vi "Dialog window display loop.vi"(1 "Loop ID":T1, 11 "error in (no error)":errorcluster) -> ()   [LabVIEW 2011]
uses:
  Application Structure/Loop ID.ctl
  Application Structure/QSM State List.ctl
  emi cndiates/E&S/reate/S&E Event source.ctl
  Annotation/Annotation Message.ctl
  emi Lib/System 01/0 - General/emi_Read System ID.vi
  emi Lib/System 01/0 - General/App/Loop control 2/Private/_emi_ SMLoop start condition.vi
  emi Lib/System 01/0 - General/App/Loop control 2/Private/_emi_ SMLoop Error Check.vi
  emi Lib/Basic/0 - General/Error/emi_Is Error.vi
  emi Lib/System 01/0 - General/App/Loop control 2/Private/_emi_SMLoop Register new.vi
  emi Lib/System 01/0 - General/S&E reporting/emi_Send S&E Error message.vi
  emi Lib/Basic/0 - General/Error/emi_ Is Error state.vi
  emi Lib/System 01/0 - General/App/Loop control/Private/_emi_GFV Loop Linking.vi
  emi Lib/System 01/0 - General/App/Loop control/Private/_emi_GFV Loop Enable.vi
  emi Lib/System 01/0 - General/App/Loop control 2/Private/_emi_ SMLoop Restart.vi
  emi Lib/System 01/0 - General/App/Private/_emi_GFV App Close.vi
  emi Lib/System 01/0 - General/App/Loop control 2/Private/_emi_ SMLoop Restart Counter.vi
  emi Lib/System 01/0 - General/App/Loop control/Private/_emi_GFV Loop Running.vi
  emi Lib/System 01/0 - General/Private/_emi_GFV System ID.vi
  emi Lib/System 01/0 - General/S&E reporting/Private/_emi_S&E Q Generator.vi
  <vilib>/Utility/error.llb/Clear Errors.vi
  emi Lib/System 01/0 - General/App/Loop control/Private/_emi_GFV stop a loop so it can reset.vi
  emi Lib/System 01/1 - GUI/Profiling Mar-In/Splash & About/Private/emi_Splash&About Screen.vi
  Application Structure/QSM/QSM Q holder.vi
  emi Lib/Basic/0 - General/Time/Private/emi_Time offset holder.vi
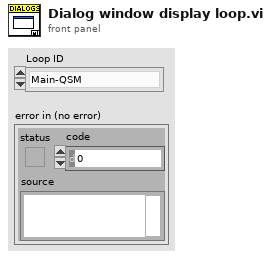
[diagram p1: front panel]
types:
  T1 = typedef "Loop ID.ctl" = enum16{"Main-QSM", "Main-Dialog", "Main-Ind Upd", "Main-Graph Upd", "Main-Debug", "Main-DebugW1", "Main-DebugW2", "Main-SE Handler", "Interface-PCP", "Interface-CANbus", "Interface-Modem", "Var Handling-Beat", "Var Handling-From PCP", "Var Handling-File storage", "Var Handling-From Simulator", "GUI-GrphW Mast", "GUI-GrphW Slav", "SIM-Tool W1", "SIM-Tool W2", "Alm-Sound", "LEIN-motor", "Tool data gatherer Qer", "Tool Data LEIN STAT2 dekoder", "Indicator Value Update", "Tool STAT2 dedicated reader", "Tool ID handler", "Detail View L1", "Detail View L2", "Main display enable view", "Sequence runner", "Voltage setpoint", "Resistance setpoint", "Stroker Wizard L1", "Stroker Wizard L2", "Alarm Handling", "Annotations Tip Strip", "Magna Interface", "Modem Status", "Var Handling - Modem Status", "Power interface detector"}
  T2 = typedef "QSM State List.ctl" = enum16{"Idle", "Init <<<Start>>>", "Init Reg Controlers", "Init Stroker Ref FGV", "Init Driller Ref FGV", "Init Tractor Ref FGV", "Init All loops", "Init Mem Ctls", "Init GUI", "Init<<<End>>>", "Show options", "Options updated", "Show User Dialog", "User Updated", "Show About", "Show Help", "Debug Visibility", "End Application", "Mem Ctls", "Mem Graphs", "Post", "-------------", "Dialog Common Analog", "Chart Init", "Chart Var Selector Rings init", "Chart Read Settings from INI", "Chart Clear", "Chart Selection Changed", "Chart Time Changed", "Graph Dialog Show", "Annotation, New", "Annotation Created", "PCP CMD", "Show Welcome screen", "Dialog Tool analog", "Update PCP resistance", "Tool CMD", "Chart single autoscale", "Tool connenction state", "Show detailed view", "Sequences updated", "Show stroker wizard", "Change tool", "Reset Telemetry", "Update control units", "Stop Logging", "Start New Loggfile", "Log Init", "Copy INI files"}
  T3 = typedef "S&E Event source.ctl" = enum16{"User", "Instrument", "Application", "Windows"}
  T4 = typedef "Annotation Message.ctl" = cluster{"Annotation":string, "User":string, "time":timestamp}
  T5 = typedef "_emi_ SMLoop sates.ctl" = enum16{"Init", "Standby", "Start", "Normal Operation", "Stop", "Error Handling", "End", "Post"}
  T6 = cluster{"Placeholder":bool, "Dialog Selector Q":refnum<queue>}
  T7 = typedef "Dialog selection cluster.ctl" = cluster{"ID":T8, "Details":variant}
  T8 = typedef "Dialog box ID.ctl" = enum16{"About dialog Box", "Options dialog box", "User dialog Box", "Custom dialog...", "Variables Common Analog", "Annotation", "Welcome screen", "Variables Tool Analog", "High G graph display", "Sequence setup", "Unused"}
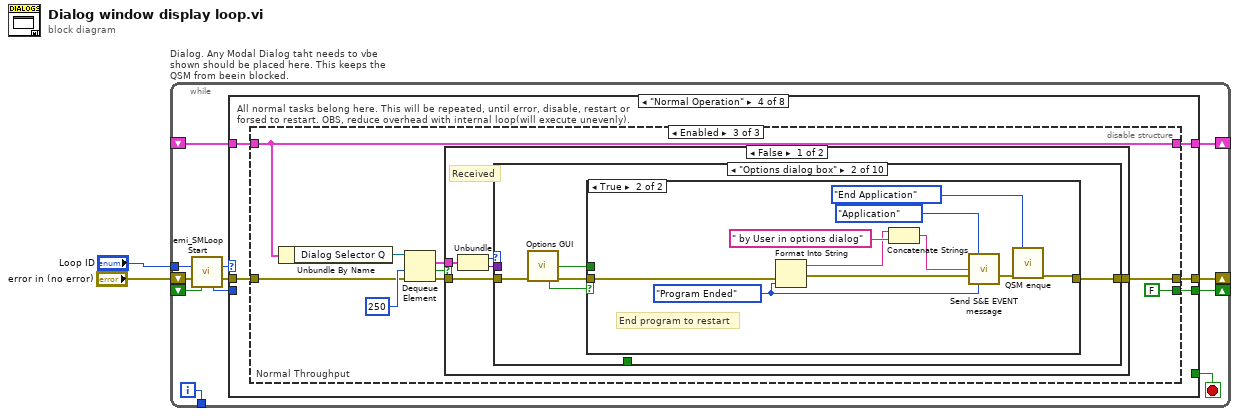
[diagram p0: block diagram]
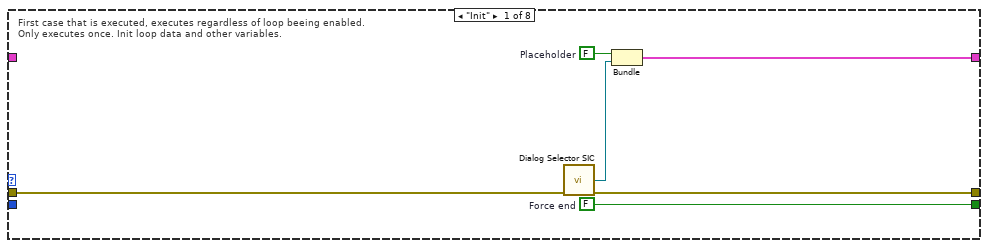
[diagram p2: hidden frame]
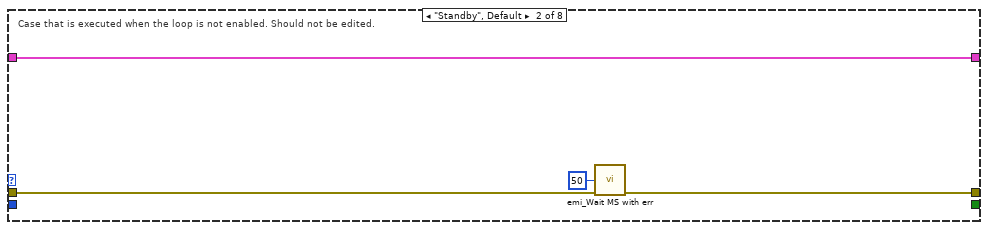
[diagram p3: hidden frame]
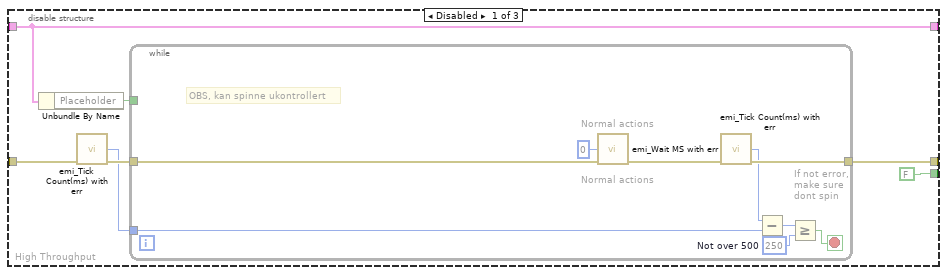
[diagram p5: hidden frame]
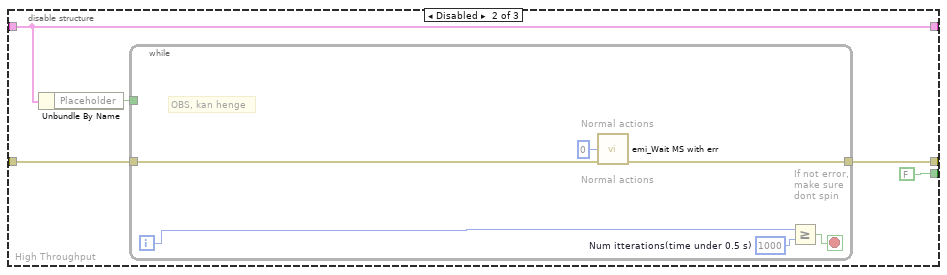
[diagram p6: hidden frame]
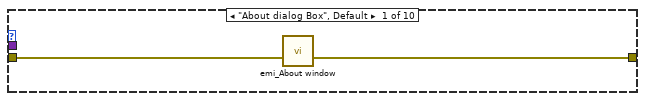
[diagram p7: hidden frame]
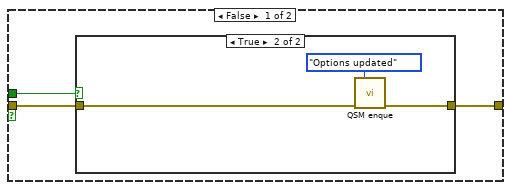
[diagram p8: hidden frame]
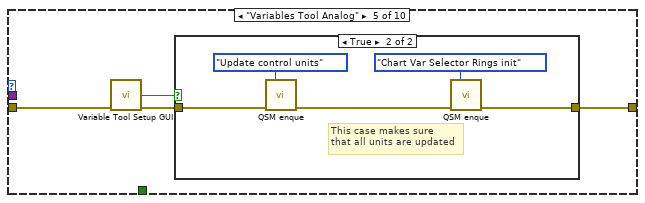
[diagram p12: hidden frame]
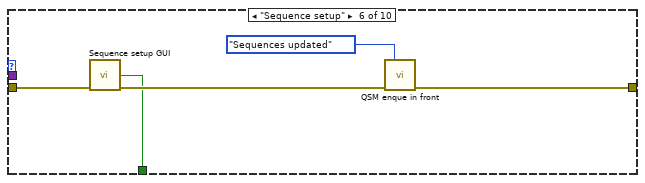
[diagram p14: hidden frame]
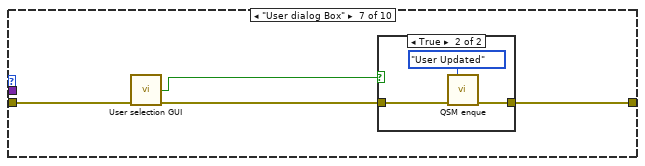
[diagram p15: hidden frame]
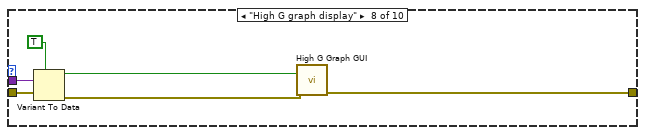
[diagram p17: hidden frame]
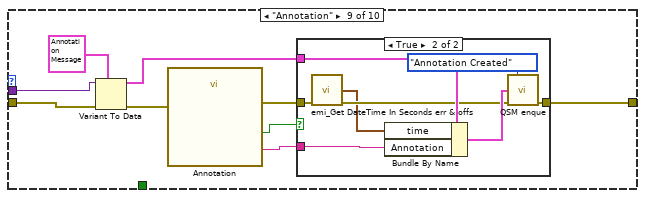
[diagram p18: hidden frame]
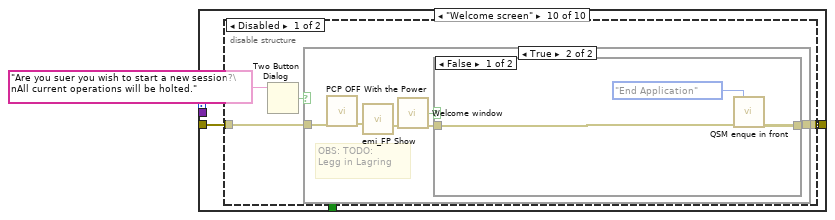
[diagram p20: hidden frame]
diagram:
  n1 = while "Dialog. Any Modal Dialog taht needs to vbe shown should be placed here. This keeps the QSM from beein blocked." {
    shift-right: [w14] -> _
    shift-left: _ -> [w10]
    shift-right: [w12] -> _
    shift-left: "error in (no error)" -> [w8]
    tunnel: [w11] -> _
    shift-right: [w9] -> _
    shift-left: _ -> [w5]
    tunnel: "Loop ID" -> [w6]
    i -> [w11]
    stop <- w13 stop-if-true
    n2 = call "emi_SMLoop Start.vi"("Loop ID"=w6, "error in (no error)"=w8, "Force Stop(F)"=w5) -> ("Loop command"=w4:T5, "error out"=w7:errorcluster, "Loop ID out"=w3:i32)  [unwired: 10 in]
    n3 = case shown="\"Normal Operation\"" w4 {
      tunnel: [w20 w21 w25 w29 w181 w184 w185 w188] -> w14
      tunnel: [_ _ _ _ _ _ _ TRUE] -> w13
      tunnel: w7 -> [w17 w23 w26 w31 w182 w183 w186 w189]
      tunnel: [w16 w22 w26 w30 w182 w183 w186 w189] -> w12
      tunnel: w10 -> [_ w21 w25 w28 w181 w184 w185 w188]
      tunnel: [w18 _ _ w27 _ _ _ _] -> w9
      tunnel: w3 -> [_ _ _ _ _ _ _ _]
      frame "Init" {
        w18 = FALSE  # Force end
        w19 = FALSE  # Placeholder
        # "First case that is executed, executes regardless of loop beeing enabled.\nOnly executes once. Init loop data and other variables."
        n4 = call "Dialog Selector SIC.vi"("error in (no error)"=w17) -> ("Dialog Selector Q"=w15:refnum<queue>, "error out"=w16:errorcluster)  [unwired: 13 in]
        n5 = Bundle("Placeholder"=w19, "Dialog Selector Q"=w15) -> (w20:T6)  [unwired: 1 in]
      }
      frame "Standby", Default {
        # "Case that is executed when the loop is not enabled. Should not be edited."
        n6 = call "emi_Wait MS with err.vi"("milliseconds to wait(0)"=u32 50, "error in (no error)"=w23) -> ("error out"=w22:errorcluster)  [unwired: 13 in]
      }
      frame "Start" {
        # "Start or restart the loop. Should perform any init code. Open channel and so on. \nWill perform each time the system is restarted."
      }
      frame "Normal Operation" {
        # "All normal tasks belong here. This will be repeated, until error, disable, restart or\nforsed to restart. OBS, reduce overhead with internal loop(will execute unevenly)."
        n7 = disable-structure shown="Enabled" {
          disable-tunnel: w31 -> [w35 w48 w64]
          disable-tunnel: [w37 w51 w59] -> w30
          disable-tunnel: [w38 w52 w66] -> w29
          disable-tunnel: w28 -> [w38 w52 w66]
          disable-tunnel: [FALSE ("Force End") FALSE ("Force End") FALSE ("Force End")] -> w27
          frame Disabled {
            # "High Throughput"
            n8 = Unbundle By Name(w38) -> ("Placeholder"=w36:bool)
            n9 = call "emi_Tick Count(ms) with err.vi"("error in (no error)"=w35) -> ("millisecond timer value"=w33:u32, "error out"=w34:errorcluster)  [unwired: 13 in]
            n10 = while {
              tunnel: w34 -> [w41]
              tunnel: [w47] -> w37
              tunnel: w36 -> [_]
              tunnel: w33 -> [w46]
              stop <- w40 stop-if-true
              w43 = u32 250  # Not over 500
              # "OBS, kan spinne ukontrollert"
              # "If not error,\nmake sure \ndont spin"
              # "Normal actions"
              # "Normal actions"
              n11 = call "emi_Wait MS with err.vi"("milliseconds to wait(0)"=u32 0, "error in (no error)"=w41) -> ("error out"=w42:errorcluster)  [unwired: 13 in]
              n12 = call "emi_Tick Count(ms) with err.vi"("error in (no error)"=w42) -> ("millisecond timer value"=w45:u32, "error out"=w47:errorcluster)  [unwired: 13 in]
              n13 = Subtract(x=w45, y=w46) -> (x-y=w44:u32)
              n14 = Greater Or Equal?(x=w44, y=w43) -> (x >= y?=w40:bool)
            }
          }
          frame Disabled {
            # "High Throughput"
            n15 = Unbundle By Name(w52) -> ("Placeholder"=w50:bool)
            n16 = while {
              tunnel: [w54] -> w51
              tunnel: w50 -> [_]
              tunnel: w48 -> [w55]
              i -> [w53]
              stop <- w57 stop-if-true
              w58 = u32 1000  # Num itterations(time under 0.5 s)
              # "OBS, kan henge"
              # "If not error,\nmake sure \ndont spin"
              # "Normal actions"
              # "Normal actions"
              n17 = call "emi_Wait MS with err.vi"("milliseconds to wait(0)"=u32 0, "error in (no error)"=w55) -> ("error out"=w54:errorcluster)  [unwired: 13 in]
              n18 = Greater Or Equal?(x=w53, y=w58) -> (x >= y?=w57:bool)
            }
          }
          frame Enabled {
            # "Normal Throughput"
            n19 = Unbundle By Name(w66) -> ("Dialog Selector Q"=w63:refnum<queue>)
            n20 = Dequeue Element(queue=w63, timeout in ms (-1)=250, error in (no error)=w64) -> (element=w62:T7, timed out?=w61:bool, error out=w60:errorcluster)  [unwired: 1 out]
            n21 = case shown="False" w61 {
              tunnel: w60 -> [w72 w180]
              tunnel: [w68 w180] -> w59
              tunnel: w62 -> [w71 _]
              frame False {
                # "Received"
                n22 = Unbundle(w71) -> ("ID"=w70:T8, "Details"=w69:variant)
                n23 = case shown="\"Options dialog box\"" w70 {
                  tunnel: w72 -> [w74 w79 w97 w98 w102 w113 w116 w125 w135 w146]
                  tunnel: w69 -> [_ _ _ _ _ _ _ w126 w130 _]
                  tunnel: [w73 w77 w97 w98 w99 w110 w117 w127 w136 w147] -> w68
                  tunnel: [_ _ _ _ _ w109 _ _ _ _] -> _
                  frame "About dialog Box", Default {
                    n24 = call "emi_About window.vi"("error in (no error)"=w74) -> ("error out"=w73:errorcluster)  [unwired: 14 in]
                  }
                  frame "Options dialog box" {
                    n25 = call "Options GUI.vi"("error in (no error)"=w79) -> ("OK"=w76:bool, "Restart software"=w75:bool, "error out"=w78:errorcluster)  [unwired: 12 in]
                    n26 = case shown="True" w75 {
                      tunnel: w78 -> [w82 w88]
                      tunnel: [w81 w87] -> w77
                      tunnel: w76 -> [w80 _]
                      frame False {
                        n27 = case shown="True" w80 {
                          tunnel: w82 -> [w83 w86]
                          tunnel: [w83 w85] -> w81
                          frame False {
                          }
                          frame True {
                            n28 = call "QSM enque.vi"("State"=QSM_State_List."Options updated", "error in"=w86) -> ("error out"=w85:errorcluster)  [unwired: 13 in]
                          }
                        }
                      }
                      frame True {
                        w92 = enum16{"Program Started", "Program Ended"}."Program Ended" ("App Events")
                        # "End program to restart"
                        n29 = Format Into String(error in=w88, w92) -> (resulting string=w90:string, error out=w94:errorcluster)  [unwired: 2 in]
                        n30 = Concatenate Strings(w90, " by User in options dialog" ("Note(\"\")")) -> (w89:string)
                        n31 = call "Send S&E EVENT message.vi"("Event Source(user)"=S&E_Event_source."Application", "Event Description"=w89, "error in (no error)"=w94, "Loc Sub ID/Event ID(No ID)"=w92) -> ("error out"=w93:errorcluster)  [unwired: 10 in, 1 out]
                        n32 = call "QSM enque.vi"("State"=QSM_State_List."End Application", "error in"=w93) -> ("error out"=w87:errorcluster)  [unwired: 13 in]
                      }
                    }
                  }
                  frame "Custom dialog..." {
                  }
                  frame "Variables Common Analog" {
                    # "TODO: Reager på ending?"
                  }
                  frame "Variables Tool Analog" {
                    n33 = call "Variable Tool Setup GUI.vi"("error in (no error)"=w102) -> ("OK"=w101:bool, "error out"=w100:errorcluster)  [unwired: 13 in]
                    n34 = case shown="True" w101 {
                      tunnel: w100 -> [w103 w107]
                      tunnel: [w103 w106] -> w99
                      frame False {
                      }
                      frame True {
                        # "This case makes sure\nthat all units are updated"
                        n35 = call "QSM enque.vi"("State"=QSM_State_List."Update control units", "error in"=w107) -> ("error out"=w104:errorcluster)  [unwired: 13 in]
                        n36 = call "QSM enque.vi"("State"=QSM_State_List."Chart Var Selector Rings init", "error in"=w104) -> ("error out"=w106:errorcluster)  [unwired: 13 in]
                      }
                    }
                  }
                  frame "Sequence setup" {
                    n37 = call "Sequence setup GUI.vi"("error in (no error)"=w113) -> ("OK"=w109:bool, "error out"=w111:errorcluster)  [unwired: 13 in]
                    n38 = call "QSM enque in front.vi"("State"=QSM_State_List."Sequences updated", "error in"=w111) -> ("error out"=w110:errorcluster)  [unwired: 13 in]
                  }
                  frame "User dialog Box" {
                    n39 = call "User selection GUI.vi"("error in (no error)"=w116) -> ("OK"=w114:bool, "error out"=w115:errorcluster)  [unwired: 13 in]
                    n40 = case shown="True" w114 {
                      tunnel: [w118 w121] -> w117
                      tunnel: w115 -> [w118 w119]
                      frame False {
                      }
                      frame True {
                        n41 = call "QSM enque.vi"("State"=QSM_State_List."User Updated", "error in"=w119) -> ("error out"=w121:errorcluster)  [unwired: 13 in]
                      }
                    }
                  }
                  frame "High G graph display" {
                    n42 = Variant To Data(error in=w125, type=TRUE ("Show last(T)"), Variant=w126) -> (data=w123:bool, error out=w122:errorcluster)
                    n43 = call "High G Graph GUI.vi"("Show last(T)"=w123, "error in (no error)"=w122) -> ("error out"=w127:errorcluster)  [unwired: 13 in]
                  }
                  frame "Annotation" {
                    n44 = Variant To Data(error in=w135, type=T4 {"Annotation"="", "User"="", "time"=timestamp(0 s since 1904-01-01)} ("output cluster"), Variant=w130) -> (data=w129:T4, error out=w132:errorcluster)
                    n45 = call "Annotation"("error in (no error)"=w132) -> ("Annotation"=w133:string, "OK"=w128:bool, "error out"=w134:errorcluster)  [unwired: 16 in]
                    n46 = case shown="True" w128 {
                      tunnel: [w137 w145] -> w136
                      tunnel: w134 -> [w137 w140]
                      tunnel: w133 -> [_ w143]
                      tunnel: w129 -> [_ w141]
                      frame False {
                      }
                      frame True {
                        n47 = call "emi_Get DateTime In Seconds err & offs.vi"("error in (no error)"=w140) -> ("Time"=w138:timestamp, "error out"=w139:errorcluster)  [unwired: 13 in]
                        n48 = Bundle By Name(cluster=w141, "time"=w138, "Annotation"=w143) -> (w144:T4)
                        n49 = call "QSM enque.vi"("State"=QSM_State_List."Annotation Created", "Value"=w144, "error in"=w139) -> ("error out"=w145:errorcluster)  [unwired: 12 in]
                      }
                    }
                  }
                  frame "Welcome screen" {
                    n50 = disable-structure shown="Disabled" {
                      disable-tunnel: [w151 w179] -> w147
                      disable-tunnel: w146 -> [w149 w179]
                      frame Disabled {
                        n51 = Two Button Dialog(message="Are you suer you wish to start a new session?\nAll current operations will be holted.") -> (T button?=w150:bool)  [unwired: 2 in]
                        n52 = case shown="True" w150 {
                          tunnel: [w152 w156] -> w151
                          tunnel: w149 -> [w152 w154]
                          frame False {
                          }
                          frame True {
                            # "OBS: TODO:\nLegg in Lagring"
                            n53 = call "PCP OFF With the Power.vi"("error In"=w154) -> ("error out"=w153:errorcluster)  [unwired: 14 in]
                            n54 = call "emi_FP Show.vi"("error in (no error)"=w153) -> ("error out"=w158:errorcluster)  [unwired: 13 in, 1 out]
                            n55 = call "Welcome window.vi"("error in (no error)"=w158) -> ("OK"=w157:bool, "error out"=w155:errorcluster)  [unwired: 12 in, 1 out]
                            n56 = case shown="False" w157 {
                              tunnel: [w159 w162] -> w156
                              tunnel: w155 -> [w160 w163]
                              frame False {
                                n57 = call "QSM enque in front.vi"("State"=QSM_State_List."End Application", "error in"=w160) -> ("error out"=w159:errorcluster)  [unwired: 13 in]
                              }
                              frame True {
                                n58 = To Unsigned Word Integer(number=QSM_State_List."Init<<<End>>>" ("SMAct")) -> (unsigned 16bit integer=w164:u16)
                                n59 = To Unsigned Word Integer(number=QSM_State_List."Init <<<Start>>>" ("SMAct")) -> (unsigned 16bit integer=w168:u16)
                                n60 = Subtract(x=w164, y=w168) -> (x-y=w165:u16)
                                n61 = Increment(x=w165) -> (x+1=w169:u16)
                                n62 = for {
                                N: w169 -> [_]
                                tunnel: w163 -> [w178]
                                tunnel: w168 -> [w177]
                                tunnel: [w171] -> w162
                                i -> [w176]
                                n63 = To Unsigned Word Integer(number=w176) -> (unsigned 16bit integer=w174:u16)
                                n64 = Add(x=w177, y=w174) -> (x+y=w175:u16)
                                n65 = Variant To Data(error in=w178, type=QSM_State_List."Idle" ("SMAct"), Variant=w175) -> (data=w170:T2, error out=w172:errorcluster)
                                n66 = call "QSM enque.vi"("State"=w170, "error in"=w172) -> ("error out"=w171:errorcluster)  [unwired: 13 in]
                                }
                              }
                            }
                          }
                        }
                      }
                      frame Enabled {
                      }
                    }
                  }
                }
              }
              frame True {
                # "Timeout"
              }
            }
          }
        }
      }
      frame "Stop" {
        # "Stop the loop. May be restarted later. Close interfaces and the like"
      }
      frame "Error Handling" {
        # "Loop automaticaly returns here after error is found. If error is cleared, Loop wil continue\nas normal(if was operative when error."
      }
      frame "End" {
        # "Only executes at application end has. Should performa any action the loop needs to finnish. \nExecutes only once."
      }
      frame "Post" {
      }
    }
  }
